vi "Read Image File (ARGB).vi"(7 "Image Read Size (Default: FULL_SIZE)":T1, 8 "error in (no error)":errorcluster, 10 "ARGB Image Destination in":T2, 11 "Filepath":path) -> (0 "error out":errorcluster, 3 "ARGB Image Destination":T2)   [LabVIEW 2020, in "image.lvlib"]
doc: "Read an Image file. A broad range of file formats are supported including jpeg, bitmap, png, webp, tiff and others."
uses:
  image.lvlib
  ARGB Image.ctl
  Image Read Size.ctl
  2358f293-6357-4b7a-bec3-c4e4d03be6e5.vi
  <vilib>/Utility/error.llb/Error Cluster From Error Code.vi
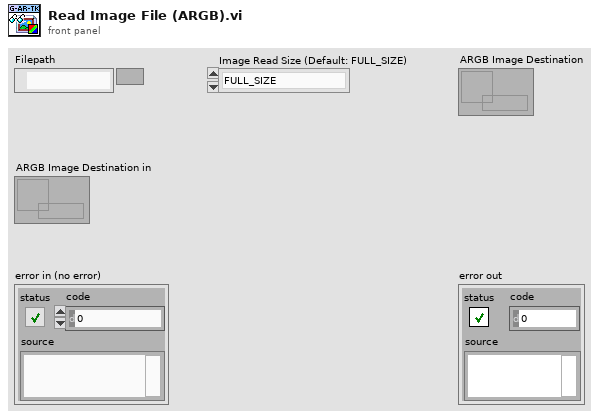
[diagram p1: front panel]
types:
  T1 = typedef "image.lvlib/Image Read Size.ctl" = enum8{"FULL_SIZE", "REDUCED_2", "REDUCED_4", "REDUCED_8"}
  T2 = typedef "image.lvlib/ARGB Image.ctl" = refnum<data-value>
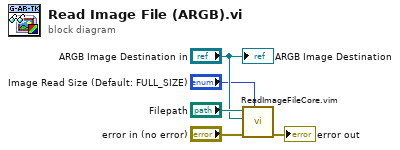
[diagram p0: block diagram]
diagram:
  n1 = call "ReadImageFileCore.vim"("Image Read Size"="Image Read Size (Default: FULL_SIZE)", "error in (no error)"="error in (no error)", "Dst"="ARGB Image Destination in", "Filepath"="Filepath") -> ("error out"=→"error out":errorcluster)  [unwired: 7 in]
  "ARGB Image Destination" <- "ARGB Image Destination in"
